vi "Destroy UserEvents.vi"(8 "error in (no error)":errorcluster, 11 "Guardar TextoPlano in":refnum<class "Guardar TextoPlano.lvclass">) -> (0 "error out":errorcluster, 3 "Guardar TextoPlano out":refnum<class "Guardar TextoPlano.lvclass">)   [LabVIEW 2020, in "Guardar TextoPlano.lvlib" / "Guardar TextoPlano.lvclass"]
uses:
  Guardar TextoPlano.lvclass
  Guardar TextoPlano.lvclass/Guardar TextoPlano.ctl
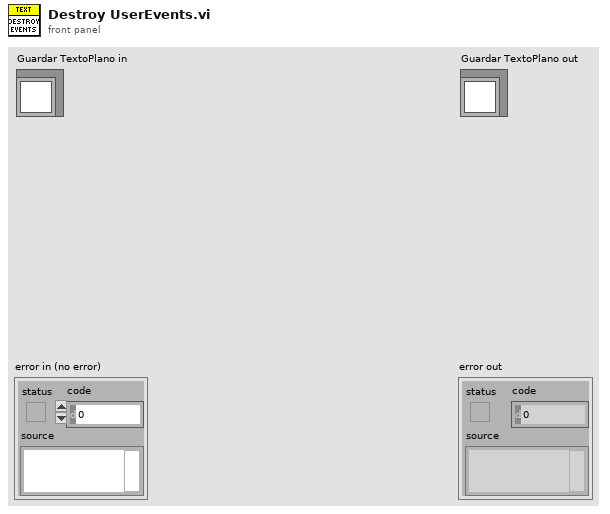
[diagram p1: front panel]
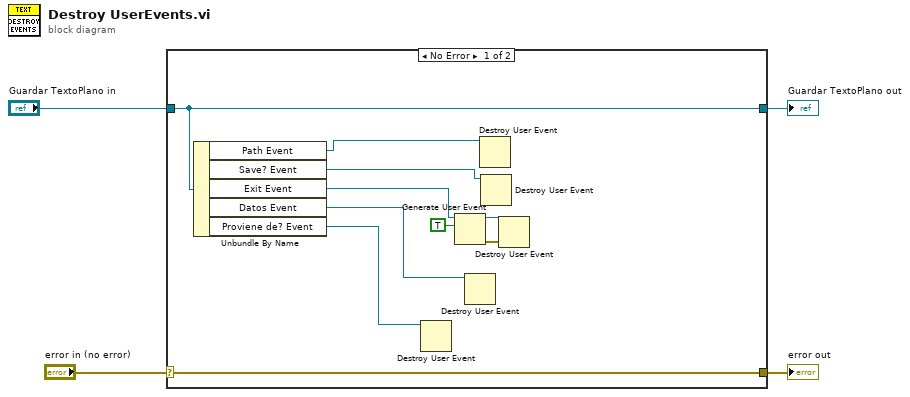
[diagram p0: block diagram]
diagram:
  n1 = case shown="No Error" "error in (no error)" {
    selector: "error in (no error)" -> [w14 w16]
    tunnel: [w14 w16] -> w3
    tunnel: [w13 w15] -> w1
    tunnel: "Guardar TextoPlano in" -> [w13 w15]
    frame No Error {
      n2 = Unbundle By Name(w13) -> ("Path Event"=w12:refnum<user-event>, "Save? Event"=w11:refnum<user-event>, "Exit Event"=w10:refnum<user-event>, "Datos Event"=w6:refnum<user-event>, "Proviene de? Event"=w5:refnum<user-event>)
      n3 = Destroy User Event(user event=w5) -> ()  [unwired: 1 in, 1 out]
      n4 = Generate User Event(user event=w10, event data cluster=TRUE ("event data")) -> (user event out=w8:refnum<user-event>, error out=w7:errorcluster)  [unwired: 2 in]
      n5 = Destroy User Event(user event=w6) -> ()  [unwired: 1 in, 1 out]
      n6 = Destroy User Event(user event=w12) -> ()  [unwired: 1 in, 1 out]
      n7 = Destroy User Event(user event=w11) -> ()  [unwired: 1 in, 1 out]
      n8 = Destroy User Event(user event=w8, error in=w7) -> ()  [unwired: 1 out]
    }
    frame Error {
    }
  }
  "error out" <- w3
  "Guardar TextoPlano out" <- w1
